vi "IsVIRunning.vi"(8 "error in (no error)":errorcluster, 10 "name or relative path":string="FrontPanel\\SICM.vi") -> (0 "error out":errorcluster, 1 "RunningVI?":bool)   [LabVIEW 2016]
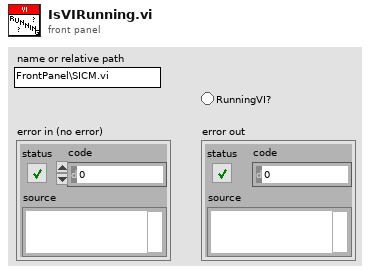
[diagram p1: front panel]
types:
  T1 = enum32{"Bad", "Idle", "Run top level", "Running"}
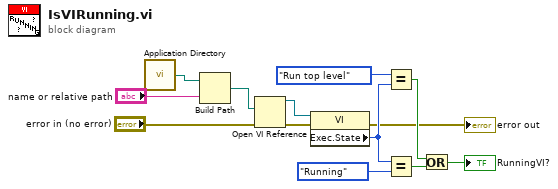
[diagram p0: block diagram]
diagram:
  n1 = call <vilib>:"Application Directory.vi"() -> ("Application Directory"=w2:path)
  n2 = Build Path(base path=w2, name or relative path="name or relative path") -> (appended path=w3:path)
  n3 = Open VI Reference(vi path=w3, error in (no error)="error in (no error)") -> (vi reference=w5:refnum<vi>, error out=w6:errorcluster)  [unwired: 4 in]
  n4 = property class="VI"(reference=w5, error in=w6) -> (error out=→"error out":errorcluster, "Exec.State"=w12:T1)  [unwired: 1 out]
  n5 = Equal?(x=T1."Run top level" ("Execution:State"), y=w12) -> (x = y?=w10:bool)
  n6 = Equal?(x=w12, y=T1."Running" ("Execution:State")) -> (x = y?=w11:bool)
  n7 = Or(x=w10, y=w11) -> (x .or. y?=→"RunningVI?":bool)
